vi "TrackingSettings.vi"(8 "error in":errorcluster, 11 "Settings In":T4={"Harware Configuration"={"Camera"="cam1", "Frames Per Second"=15, "Simulate Recording"=FALSE, "Simulated Recording Sample"=path "", "Timestamp Method"=enum."Camera Timestamp"}, "Base Recording Path"=path "", "Type Of Recording"="", "Recording Codec"="", "TrackingSettings"={"Max Radius"=0, "Threshold"=160.0, "ROI"={"Left"=0, "Top"=0, "Right"=0, "Bottom"=0, "Rotation"=0.0}}, "Calibration"={"Pixel Width (X)"=1.0, "Pixel Height (Y)"=1.0}, "Broadcast Length"=0} {"Broadcast Length" min=0; "TrackingSettings"."ROI"."Rotation" format="%.2f"; "TrackingSettings"."ROI"."Left" scale=0.0..1024.0; "TrackingSettings"."ROI"."Right" scale=0.0..1024.0; "TrackingSettings"."Threshold" scale=0.0..255.0}) -> (0 "error out":errorcluster, 2 "Canceled?":bool, 3 "Settings Out":T4={"Harware Configuration"={"Camera"="cam1", "Frames Per Second"=15, "Simulate Recording"=FALSE, "Simulated Recording Sample"=path "", "Timestamp Method"=enum."Camera Timestamp"}, "Base Recording Path"=path "", "Type Of Recording"="", "Recording Codec"="", "TrackingSettings"={"Max Radius"=0, "Threshold"=160.0, "ROI"={"Left"=0, "Top"=0, "Right"=0, "Bottom"=0, "Rotation"=0.0}}, "Calibration"={"Pixel Width (X)"=1.0, "Pixel Height (Y)"=1.0}, "Broadcast Length"=0} {"Broadcast Length" min=0; "TrackingSettings"."ROI"."Rotation" format="%.2f"; "TrackingSettings"."ROI"."Left" scale=0.0..1024.0; "TrackingSettings"."ROI"."Right" scale=0.0..1024.0; "TrackingSettings"."Threshold" scale=0.0..255.0})   [LabVIEW 2017, in "ImageAcquisitionLibrary.lvlib"]
uses:
  ImageAcquisitionLibrary.lvlib
  Settings/Settings.ctl
  <vilib>/userdefined/High Color/IMAQdx.ctl
  TrackingSettings.ctl
  Settings/Calibration.ctl
  <vilib>/Utility/error.llb/DialogType.ctl
  ImageNotifier.vi
  <vilib>/vision/NI_Vision_Development_Module.lvlib
panel:
  in  "ROI":bool
  out "Waveform Graph":u32[](graph)
  in  "TrackingSettings":T1={"Max Radius"=0, "Threshold"=255.0, "ROI"={"Left"=0, "Top"=0, "Right"=0, "Bottom"=0, "Rotation"=0.0}} {"ROI"."Rotation" format="%.2f"; "ROI"."Left" scale=0.0..1024.0; "ROI"."Right" scale=0.0..1024.0; "Threshold" scale=0.0..255.0}
  in  "OK":bool
  in  "Cancel":bool
  out "Image":T3(plugin-control)
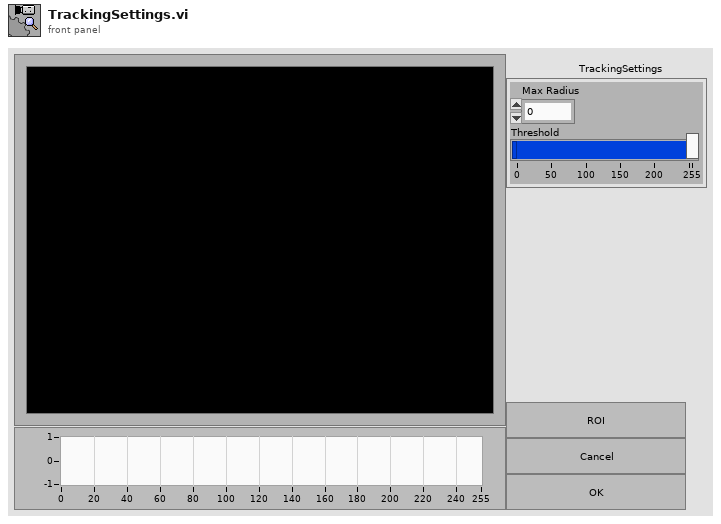
[diagram p1: front panel]
types:
  T1 = typedef "ImageAcquisitionLibrary.lvlib/TrackingSettings.ctl" = cluster{"Max Radius":i32, "Threshold":sgl, "ROI":T2}
  T2 = typedef "IMAQ Rectangle" = cluster{"Left":i32, "Top":i32, "Right":i32, "Bottom":i32, "Rotation":dbl}
  T3 = typedef "IMAQ Image.ctl" = refnum<image>
  T4 = typedef "ImageAcquisitionLibrary.lvlib/Settings.ctl" = cluster{"Harware Configuration":cluster{"Camera":T5, "Frames Per Second":u32, "Simulate Recording":bool, "Simulated Recording Sample":path, "Timestamp Method":enum16{"System Timestamp", "Camera Timestamp", "IMAQdx Timestamp"}}, "Base Recording Path":path, "Type Of Recording":string, "Recording Codec":string, "TrackingSettings":T1, "Calibration":T6, "Broadcast Length":i32}
  T5 = typedef "IMAQdx.ctl" = refnum<k21>
  T6 = typedef "ImageAcquisitionLibrary.lvlib/Calibration.ctl" = cluster{"Pixel Width (X)":dbl, "Pixel Height (Y)":dbl}
  T7 = typedef "Image Type" = u32
  T8 = typedef "ImageAcquisitionLibrary.lvlib/TrackingImages.ctl" = cluster{"Working Image":T3, "ROI Mask":T3, "Centroid Mask":T3}
  T9 = typedef "ImageAcquisitionLibrary.lvlib/AcquireData.ctl" = cluster{"Frame Data":cluster{"Image":u32[][], "Timestamp":timestamp, "Image Type":T7, "Dropped Frames":u32}, "Tracking Data":cluster{"Positions":dbl[][], "Timestamp":timestamp}, "Tracked?":bool}
  T10 = cluster{"histogram":u32[], "Minimal Value":sgl, "Maximal Value":sgl, "Starting Value":sgl, "Interval Width":sgl, "Mean Value":sgl, "Standard  Variation":sgl, "Area (pixels)":i32}
  T11 = typedef "ImageAcquisitionLibrary.lvlib/MarkersArray.ctl" = T12[]
  T12 = typedef "ImageAcquisitionLibrary.lvlib/Marker.ctl" = cluster{"X":dbl, "Color":u32, "Y ":dbl, "Owner":u8}
  T13 = cluster{"Left":dbl, "Top":dbl, "Right":dbl, "Bottom":dbl, "Rotation":dbl}
  T14 = cluster{"Left":i32, "Top":i32, "Right":i32, "Bottom":i32, "Rotation":i32}
  T15 = typedef "DialogType.ctl" = u16
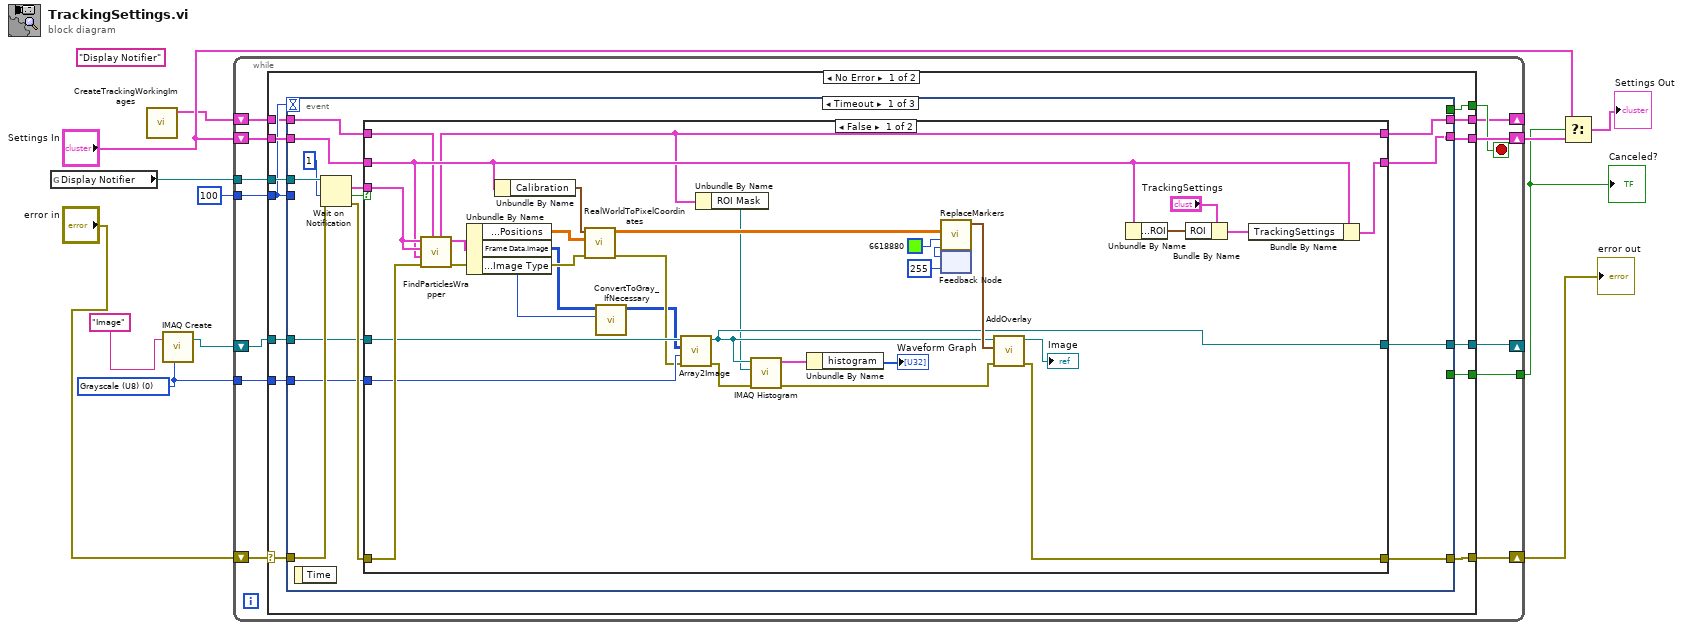
[diagram p0: block diagram]
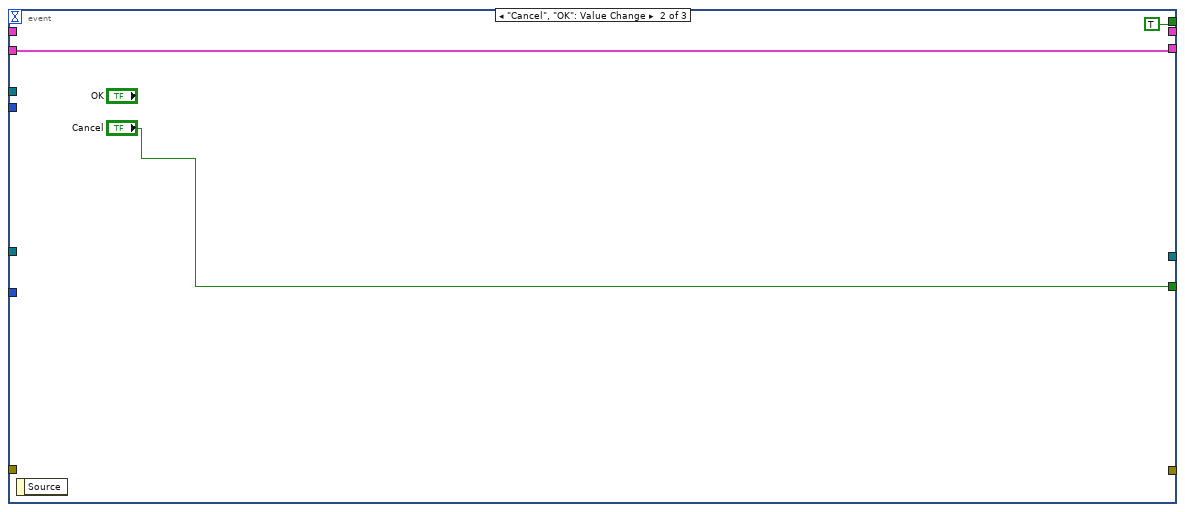
[diagram p3: hidden frame]
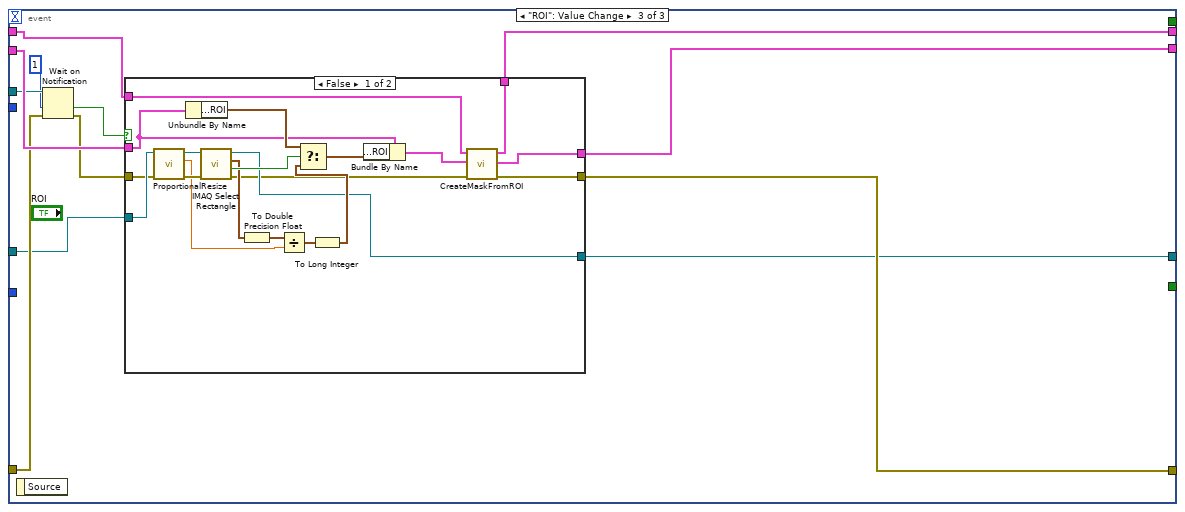
[diagram p4: hidden frame]
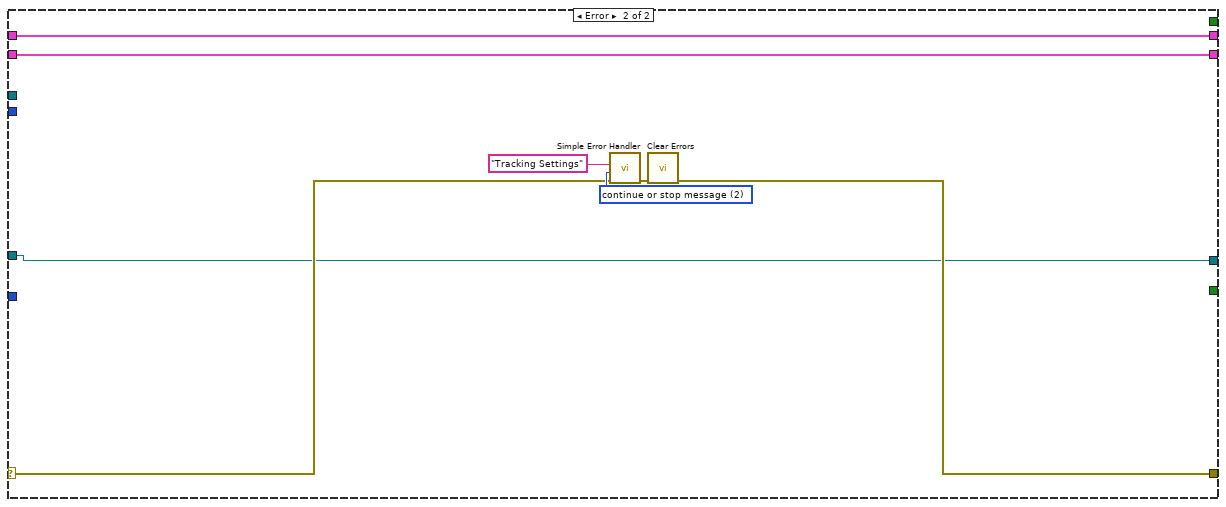
[diagram p6: hidden frame]
diagram:
  w3 = T7 0 items=["Grayscale (U8)", "Grayscale (I16)", "Grayscale (SGL)", "Complex (CSG)", "RGB (U32)", "HSL (U32)", "RGB (U64)", "Grayscale (U16)"] ("Image Type")
  (unwired) "Display Notifier" ("name (unnamed)")
  n1 = global read "ImageNotifier.vi" "Display Notifier"() -> (w1:refnum<notifier>)
  n2 = call "CreateTrackingWorkingImages.vi"() -> ("Tracking Images"=w4:T8)  [unwired: 10 in, 1 out]
  n3 = call "IMAQ Create"("Image Name"="Image", "Image Type"=w3) -> ("New Image"=w5:T3)  [unwired: 3 in, 1 out]
  n4 = while {
    shift-right: [w25] -> w12
    shift-left: "Settings In" -> [w23]
    shift-right: [w24] -> w9
    shift-left: "error in" -> [w18]
    tunnel: [w20] -> w7
    tunnel: w1 -> [w22]
    tunnel: 100 ("timeout in ms (-1)") -> [w21]
    shift-right: [w15] -> _
    shift-left: w5 -> [w17]
    tunnel: w3 -> [w14]
    shift-right: [w13] -> _
    shift-left: w4 -> [w16]
    stop <- w19 stop-if-true
    n5 = case shown="No Error" w18 {
      selector: w18 -> [w31 w133]
      tunnel: [w38 w131] -> w25
      tunnel: [w37 w132] -> w24
      tunnel: w23 -> [w36 w131]
      tunnel: w22 -> [w35 _]
      tunnel: w21 -> [w34 _]
      tunnel: [w33 _] -> w20
      tunnel: [w32 _] -> w19
      tunnel: w17 -> [w30 w130]
      tunnel: w16 -> [w29 w129]
      tunnel: [w28 w130] -> w15
      tunnel: w14 -> [w27 _]
      tunnel: [w26 w129] -> w13
      frame No Error {
        n6 = event shown="[0] Timeout" {
          selector: _ -> [_ _ _]
          dyn-events: _ -> [_ _ _]
          timeout: w34 -> [_ _ _]
          tunnel: [w52 w90 w102] -> w38
          tunnel: [w51 _ w104] -> w37
          tunnel: w36 -> [w50 w90 w103]
          tunnel: w35 -> [w49 _ w101]
          tunnel: w34 -> [_ _ _]
          tunnel: w31 -> [w48 _ w100]
          tunnel: [_ "Cancel" _] -> w33
          tunnel: [_ TRUE _] -> w32
          tunnel: w30 -> [w43 _ w96]
          tunnel: w29 -> [w42 _ w94]
          tunnel: [w41 _ w95] -> w28
          tunnel: w27 -> [w40 _ _]
          tunnel: [w39 _ w93] -> w26
          event Timeout {
            n7 = event-data() -> ()  [unwired: 1 in, 1 out]
            n8 = Wait on Notification(notifier=w49, timeout in ms (-1)=1, error in (no error)=w48) -> (notification=w46:T9, timed out?=w45:bool, error out=w47:errorcluster)  [unwired: 1 in, 1 out]
            n9 = case shown="False" w45 {
              tunnel: [w85 w89] -> w52
              tunnel: [w62 w88] -> w51
              tunnel: w50 -> [w60 w89]
              tunnel: w47 -> [w83 w88]
              tunnel: w46 -> [w81 _]
              tunnel: w43 -> [w71 w87]
              tunnel: w42 -> [w57 w86]
              tunnel: [w65 w87] -> w41
              tunnel: w40 -> [w70 _]
              tunnel: [w56 w86] -> w39
              frame False {
                n10 = call "FindParticlesWrapper.vi"(7:w57, "error in"=w83, "Settings"=w60, "Data Old"=w81, "Data"=w81) -> ("error out"=w58:errorcluster, "Data Out"=w84:T9, 5:w56:T8)  [unwired: 4 in]
                n11 = Unbundle By Name(w84) -> ("Tracking Data.Positions"=w68:dbl[][], "Frame Data.Image"=w54:u32[][], "Frame Data.Image Type"=w53:T7)
                n12 = Unbundle By Name(w60) -> ("Calibration"=w67:T6)
                n13 = call "RealWorldToPixelCoordinates.vi"("error in (no error)"=w58, "Real World Points"=w68, "Calibration 2"=w67) -> ("error out"=w59:errorcluster, "Pixels"=w76:dbl[][])  [unwired: 6 in]
                n14 = call "ConvertToGray_IfNecessary.vi"("Image Type"=w53, "Image in"=w54) -> ("Image out"=w55:u32[][])  [unwired: 9 in]
                n15 = call "Array2Image.vi"("error in (no error)"=w59, "Image Type"=w70, "Image Pixels (U32)"=w55, "Image 2"=w71) -> ("error out"=w66:errorcluster, "Image"=w65:T3)  [unwired: 6 in]
                n16 = Unbundle By Name(w56) -> ("ROI Mask"=w61:T3)
                n17 = call "IMAQ Histogram"("error in (no error)"=w66, "Image Mask"=w61, "Image"=w65) -> ("error out"=w63:errorcluster, "Histogram Report"=w69:T10)  [unwired: 7 in]
                n18 = Unbundle By Name(w69) -> ("histogram"=→"Waveform Graph":u32[])
                n19 = feedback #1(u8 255 ("Owner Out")) -> (w73:u8)
                n20 = call "ReplaceMarkers.vi"("Owner"=w73, "Color"=u32 6618880, "Pixels 3"=w76) -> ("Owner Out"=w74:u8, "MarkersArray Out"=w77:T11)  [unwired: 7 in]
                n21 = feedback-in #1(w74) -> ()
                n22 = call "AddOverlay.vi"("error in (no error)"=w63, "MarkersArray"=w77, "Refnum in"=w65) -> ("error out"=w62:errorcluster, "Refnum out"=→"Image":T3)  [unwired: 7 in]
                n23 = Unbundle By Name(w60) -> ("TrackingSettings.ROI"=w78:T2)
                n24 = Bundle By Name(cluster="TrackingSettings", "ROI"=w78) -> (w79:T1)
                n25 = Bundle By Name(cluster=w60, "TrackingSettings"=w79) -> (w85:T4)
              }
              frame True {
              }
            }
          }
          event "Cancel", "OK": Value Change {
            n26 = event-data() -> ()  [unwired: 1 in, 1 out]
          }
          event "ROI": Value Change {
            n27 = event-data() -> ()  [unwired: 1 in, 1 out]
            n28 = Wait on Notification(notifier=w101, timeout in ms (-1)=1, error in (no error)=w100) -> (timed out?=w98:bool, error out=w99:errorcluster)  [unwired: 1 in, 2 out]
            n29 = case shown="False" w98 {
              tunnel: [w105 w127] -> w104
              tunnel: w103 -> [w117 w128]
              tunnel: [w109 w128] -> w102
              tunnel: w99 -> [w119 w127]
              tunnel: w96 -> [w121 w126]
              tunnel: [w111 w126] -> w95
              tunnel: w94 -> [w108 w125]
              tunnel: [w107 w125] -> w93
              frame False {
                n30 = call "ProportionalResize.vi"("error in (no error)"=w119, "Refnum in"=w121) -> ("error out"=w118:errorcluster, "Size Ratio"=w113:dbl, "Refnum out"=w120:T3)  [unwired: 7 in]
                n31 = Unbundle By Name(w117) -> ("TrackingSettings.ROI"=w124:T2)
                n32 = call "IMAQ Select Rectangle"("error in (no error)"=w118, "Image In"=w120) -> ("error out"=w106:errorcluster, "Cancelled"=w123:bool, "Rectangle"=w116:T2, "Image Out (duplicate)"=w111:T3)  [unwired: 6 in]
                n33 = To Double Precision Float(number=w116) -> (double precision float=w114:T13)
                n34 = Divide(x=w114, y=w113) -> (x/y=w112:T13)
                n35 = To Long Integer(number=w112) -> (32bit integer=w115:T14)
                n36 = Select(t=w124, s=w123, f=w115) -> (s? t:f=w122:T2)
                n37 = Bundle By Name(cluster=w117, "TrackingSettings.ROI"=w122) -> (w110:T4)
                n38 = call "CreateMaskFromROI.vi"("error in (no error)"=w106, "Settings"=w110, 11:w108) -> ("error out"=w105:errorcluster, "Settings 2"=w109:T4, "output cluster"=w107:T8)  [unwired: 6 in]
              }
              frame True {
              }
            }
          }
        }
      }
      frame Error {
        w134 = T15 2 items=["no dialog", "OK message", "continue or stop message", "OK message + warnings", "continue/stop + warnings"] ("type of dialog (OK msg:1)")
        n39 = call <vilib>:"Simple Error Handler.vi"("error source (\" \")"="Tracking Settings" ("error source (\" \")"), "type of dialog (OK msg:1)"=w134, "error in (no error)"=w133) -> ("error out"=w135:errorcluster)  [unwired: 2 in, 4 out]
        n40 = call <vilib>:"Clear Errors.vi"("error in (no error)"=w135) -> ("error out"=w132:errorcluster)  [unwired: 5 in, 1 out]
      }
    }
  }
  "error out" <- w9
  "Canceled?" <- w7
  n41 = Select(t="Settings In", s=w7, f=w12) -> (s? t:f=→"Settings Out":T4)
